vi "Motor_con.vi"(4 "Q_Process_Data_Err_IN":errorcluster caption="Q_Process_DATA_Err_IN", 6 "Q_Process_Data2_IN":refnum<queue>, 8 "Error_IN":errorcluster caption="error out", 9 "Notifier_IN":refnum<notifier>, 10 "Q_MotorCmd_Err_IN":errorcluster caption="에러 출력", 11 "Q_MotorCmd_IN":refnum<queue>) -> ()   [LabVIEW 2019]
uses:
  <vilib>/Platform/TimedLoop/XDataNode/timing_clust.ctl
  <vilib>/Platform/TimedLoop/XDataNode/nitl_modes.ctl
  <vilib>/Platform/TimedLoop/XDataNode/wakeup.ctl
  Type/SDO_Command.ctl
  CANopen/CANopen_SubVI/Controlword.ctl
  RT_GLOBAL.vi
  <vilib>/Platform/TimedLoop/XDataNode/XDataNode.xnode
  <vilib>/Platform/TimedLoop/XDataNode/XDNodeRunTimeDep.lvlib
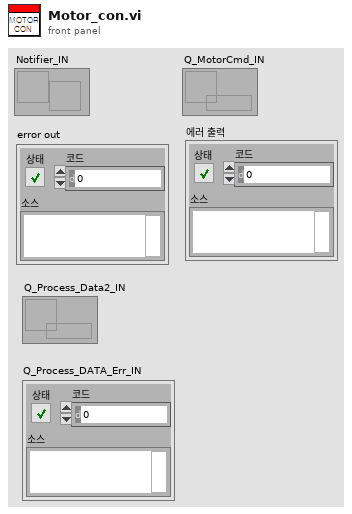
[diagram p1: front panel]
types:
  T1 = typedef "XDNodeRunTimeDep.lvlib/timing_clust.ctl" = cluster{"Expected End [f-1]":u64, "Actual End [f-1]":u64, "Finished Late? [f-1]":bool, "Expected End [i-1]":u64, "Actual End [i-1]":u64, "Finished Late? [i-1]":bool, "Expected Start [i]":u64, "Actual Start [i]":u64, "Expected Start [f]":u64, "Actual Start [f]":u64, "Source Name":string, "Structure Name":string, "Period":i64, "Deadline":i64, "Offset":i64, "Start":i64, "Priority":i32, "Timeout":i32, "Mode":T2, "Wakeup Reason":T3, "Error":errorcluster, "Source Type":string, "Secondary Source Type":string, "Global End Time":u64, "Global Start Time":u64, "Frame Duration":u64, "Iteration Duration":u64, "Assigned CPU":i32, "I/O Scan Engine Mode":u32}
  T2 = typedef "XDNodeRunTimeDep.lvlib/nitl_modes.ctl" = enum32{"No Change", "Process missed periods, maintain original phase", "Discard missed periods, maintain original phase", "Process missed periods, ignore original phase", "Discard missed periods, ignore original phase"}
  T3 = typedef "XDNodeRunTimeDep.lvlib/wakeup.ctl" = enum32{"Normal", "Aborted", "Asynchronous wakeup", "Timing source error", "Timed loop error", "Timeout"}
  T4 = cluster{"Target":i32, "Manual":u8[], "Velocity":u32, "Acc/Dec":u32}
  T5 = typedef "SDO_Command.ctl" = enum16{"Idle", "Shutdown", "Switch On", "Enable Operation", "Disable Voltage", "Quikstop", "Disable Operation", "Fault Reset", "Manual", "Statusword", "Mode of Operation", "Mode Display", "Target Position", "Position Actual Value", "Controlword_Move", "Profile Velocity", "Profile Acceleration", "Profile Deceleration", "Move"}
  T6 = typedef "CANFrameControl.ctl" = cluster{"identifier":u32, "extended?":bool, "type":u8, "payload":u8[]}
  T7 = cluster{"Cmd":string, "Data1":variant, "Data2":variant}
  T8 = typedef "Controlword.ctl" = u8
  T9 = cluster{"[0]":bool, "[1]":bool, "[2]":bool, "[3]":bool, "[4]":bool, "[5]":bool, "[6]":bool, "[7]":bool, "[8]":bool, "[9]":bool, "[10]":bool, "[11]":bool, "[12]":bool, "[13]":bool, "[14]":bool, "[15]":bool}
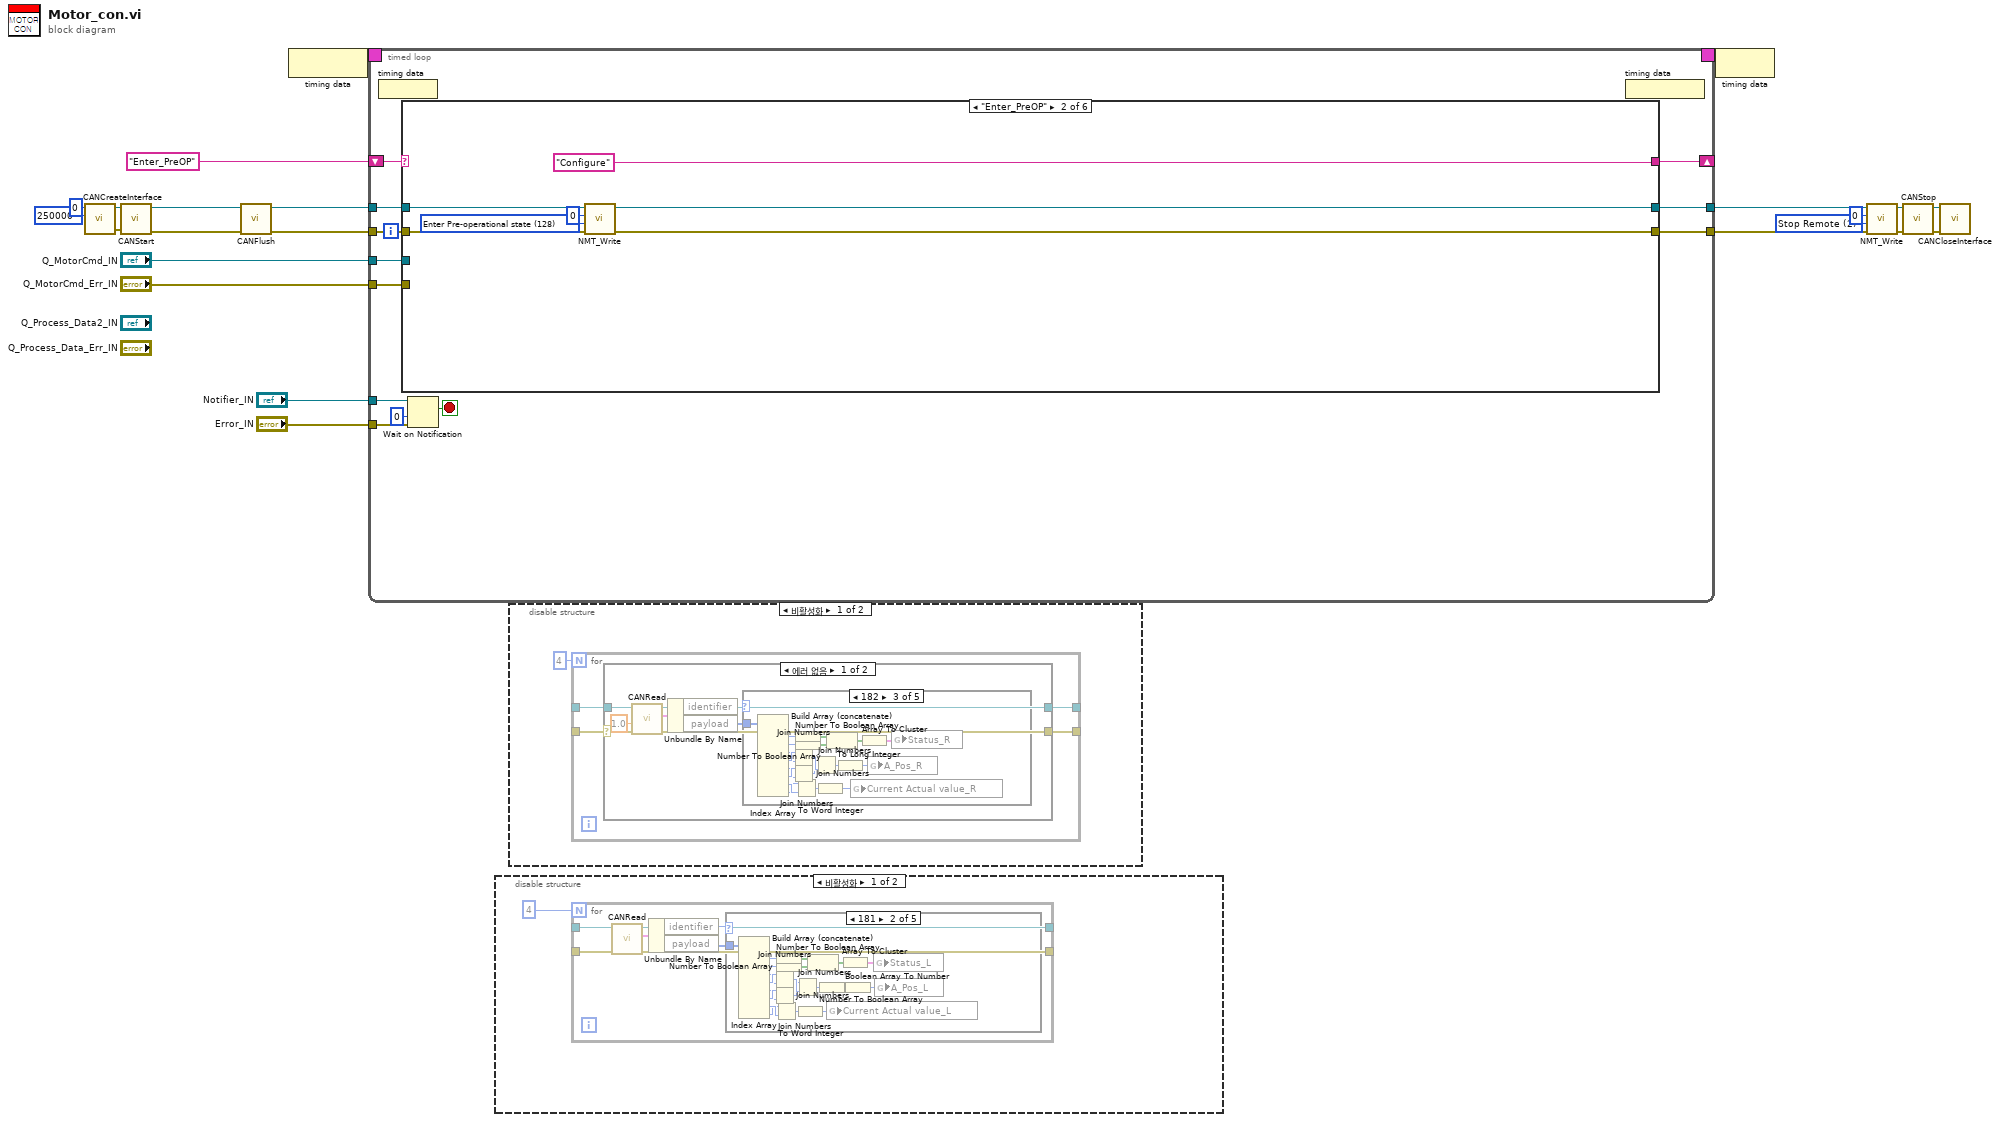
[diagram p0: block diagram]
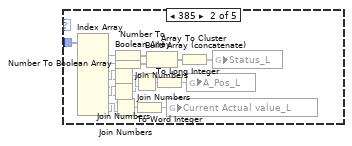
[diagram p3: hidden frame]
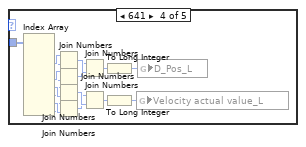
[diagram p4: hidden frame]
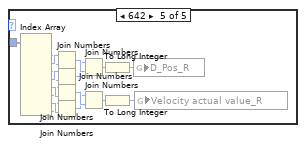
[diagram p5: hidden frame]
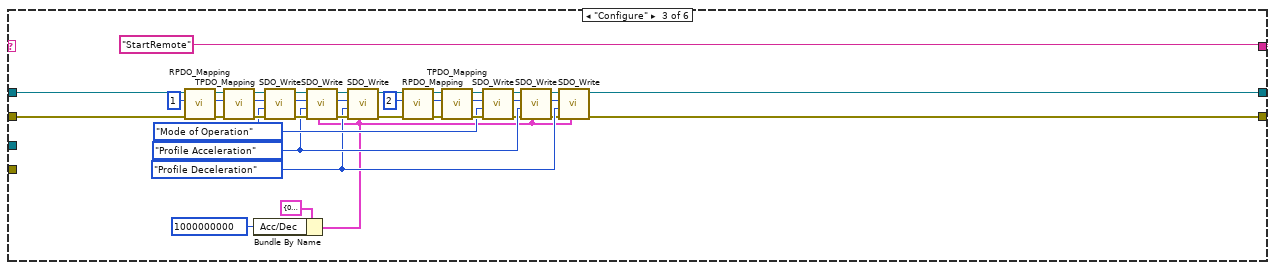
[diagram p9: hidden frame]
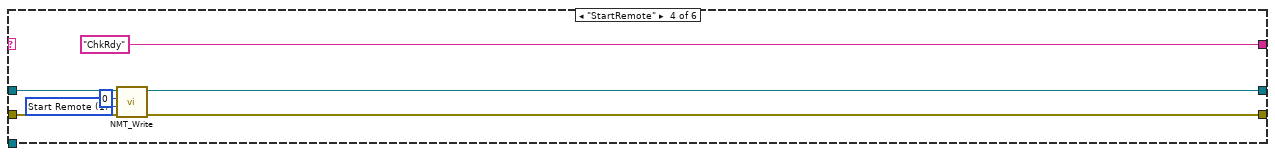
[diagram p10: hidden frame]
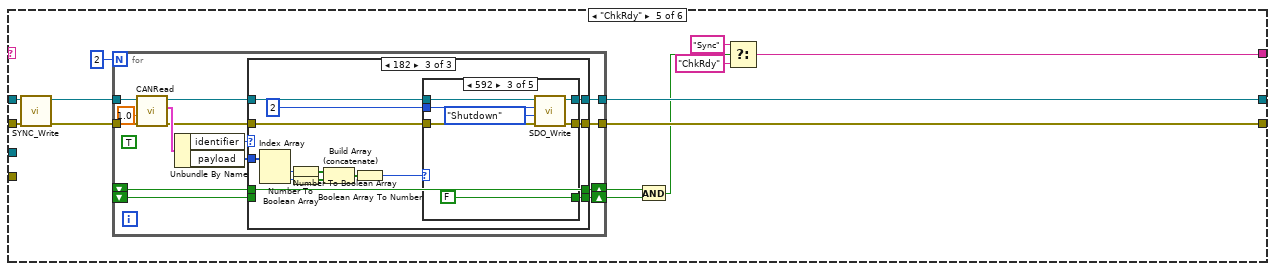
[diagram p11: hidden frame]
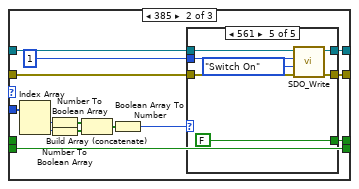
[diagram p13: hidden frame]
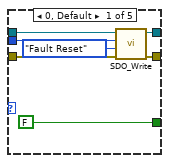
[diagram p14: hidden frame]
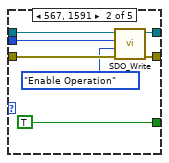
[diagram p15: hidden frame]
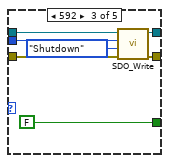
[diagram p16: hidden frame]
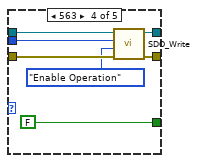
[diagram p17: hidden frame]
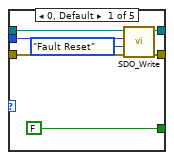
[diagram p18: hidden frame]
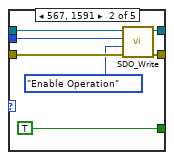
[diagram p19: hidden frame]
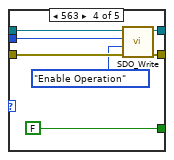
[diagram p20: hidden frame]
diagram:
  w15 = u8 2 items=["Start Remote"=1, "Stop Remote"=2, "Enter Pre-operational state"=128, "Reset node"=129, "Reset communication"=130] ("Command")
  n1 = call <vilib>:"CANCreateInterface.vi"("baud rate (125000 bps)"=u32 250000, "interface index"=u32 0) -> ("error out"=w8:errorcluster, "interface object out"=w9:refnum<k20>)  [unwired: 8 in]
  n2 = call <vilib>:"CANStart.vi"("error in (no error)"=w8, "interface object in"=w9) -> ("error out"=w3:errorcluster, "interface object out"=w4:refnum<k20>)  [unwired: 8 in]
  n3 = call <vilib>:"CANFlush.vi"("error in (no error)"=w3, "interface object in"=w4) -> ("error out"=w1:errorcluster, "interface object out"=w2:refnum<k20>)  [unwired: 8 in]
  n4 = node-c288() -> (w12:T1)
  n5 = timed-loop {
    shift-right: [w35] -> _
    shift-left: "Enter_PreOP" -> [w34]
    tunnel: "Q_MotorCmd_IN" -> [w32]
    tunnel: "Q_MotorCmd_Err_IN" -> [w31]
    tunnel: [w33] -> w23
    timing: w12 -> [_]
    timing-out: [_] -> w11
    tunnel: w1 -> [w29]
    tunnel: "Notifier_IN" -> [w25]
    tunnel: "Error_IN" -> [w24]
    tunnel: w2 -> [w28]
    tunnel: [w30] -> w17
    stop <- w27 stop-if-true
    n6 = node-c288() -> ()  [unwired: 1 in]
    n7 = case shown="\"Enter_PreOP\"" w34 {
      selector: w34 -> [w40 _ _ _ _ w219]
      tunnel: [w40 "Configure" "StartRemote" "ChkRdy" w88 w220] -> w35
      tunnel: [w39 w42 w49 w80 w92 w221] -> w30
      tunnel: w28 -> [w39 w45 w52 w83 w94 w223]
      tunnel: [w38 w41 w48 w79 w91 w215] -> w33
      tunnel: w29 -> [w38 w44 w51 w82 w93 w222]
      tunnel: w32 -> [_ _ _ _ _ w230]
      tunnel: w31 -> [_ _ _ _ _ w229]
      frame "거짓", Default {
      }
      frame "Enter_PreOP" {
        w47 = u8 128 items=["Start Remote"=1, "Stop Remote"=2, "Enter Pre-operational state"=128, "Reset node"=129, "Reset communication"=130] ("Command")
        n8 = call "NMT_Write.vi"("error in"=w44, "Command"=w47, "Node_ID"=u32 0, "interface object in"=w45) -> ("error out"=w41:errorcluster, "interface object out"=w42:refnum<k20>)  [unwired: 6 in]
      }
      frame "Configure" {
        w56 = SDO_Command."Profile Deceleration" ("Command")
        w57 = SDO_Command."Profile Acceleration" ("Command")
        w58 = u32 2 ("Node_ID")
        w69 = u32 1 ("Node_ID")
        w61 = SDO_Command."Mode of Operation" ("Command")
        n9 = call "RPDO_Mapping.vi"("error in"=w51, "Node_ID"=w69, "interface object in"=w52) -> ("error out"=w77:errorcluster, "interface object out"=w78:refnum<k20>)  [unwired: 7 in]
        n10 = call "TPDO_Mapping.vi"("error in"=w77, "Node_ID"=w69, "interface object in"=w78) -> ("error out"=w75:errorcluster, "interface object out"=w76:refnum<k20>)  [unwired: 7 in]
        n11 = Bundle By Name(cluster=T4 {"Target"=0, "Manual"=[], "Velocity"=0, "Acc/Dec"=0} ("Parameter"), "Acc/Dec"=u32 1000000000) -> (w55:T4)
        n12 = call "SDO_Write.vi"("error in"=w75, "Command"=w61, "Node_ID"=w69, "interface object in"=w76) -> ("error out"=w68:errorcluster, "interface object out"=w67:refnum<k20>)  [unwired: 6 in]
        n13 = call "SDO_Write.vi"("Parameter"=w55, "error in"=w68, "Command"=w57, "Node_ID"=w69, "interface object in"=w67) -> ("error out"=w66:errorcluster, "interface object out"=w70:refnum<k20>)  [unwired: 5 in]
        n14 = call "SDO_Write.vi"("Parameter"=w55, "error in"=w66, "Command"=w56, "Node_ID"=w69, "interface object in"=w70) -> ("error out"=w62:errorcluster, "interface object out"=w63:refnum<k20>)  [unwired: 5 in]
        n15 = call "RPDO_Mapping.vi"("error in"=w62, "Node_ID"=w58, "interface object in"=w63) -> ("error out"=w73:errorcluster, "interface object out"=w74:refnum<k20>)  [unwired: 7 in]
        n16 = call "TPDO_Mapping.vi"("error in"=w73, "Node_ID"=w58, "interface object in"=w74) -> ("error out"=w71:errorcluster, "interface object out"=w72:refnum<k20>)  [unwired: 7 in]
        n17 = call "SDO_Write.vi"("error in"=w71, "Command"=w61, "Node_ID"=w58, "interface object in"=w72) -> ("error out"=w54:errorcluster, "interface object out"=w60:refnum<k20>)  [unwired: 6 in]
        n18 = call "SDO_Write.vi"("Parameter"=w55, "error in"=w54, "Command"=w57, "Node_ID"=w58, "interface object in"=w60) -> ("error out"=w53:errorcluster, "interface object out"=w59:refnum<k20>)  [unwired: 5 in]
        n19 = call "SDO_Write.vi"("Parameter"=w55, "error in"=w53, "Command"=w56, "Node_ID"=w58, "interface object in"=w59) -> ("error out"=w48:errorcluster, "interface object out"=w49:refnum<k20>)  [unwired: 5 in]
      }
      frame "StartRemote" {
        w84 = u8 1 items=["Start Remote"=1, "Stop Remote"=2, "Enter Pre-operational state"=128, "Reset node"=129, "Reset communication"=130] ("Command")
        n20 = call "NMT_Write.vi"("error in"=w82, "Command"=w84, "Node_ID"=u32 0, "interface object in"=w83) -> ("error out"=w79:errorcluster, "interface object out"=w80:refnum<k20>)  [unwired: 6 in]
      }
      frame "ChkRdy" {
        n21 = call "SYNC_Write.vi"("error in"=w93, "interface object in"=w94) -> ("error out"=w96:errorcluster, "interface object out"=w97:refnum<k20>)  [unwired: 8 in]
        n22 = for {
          N: 2 -> [_]
          tunnel: w97 -> [w107]
          tunnel: [w104] -> w92
          tunnel: w96 -> [w106]
          tunnel: [w103] -> w91
          shift-right: [w102] -> w90
          shift-left: _ -> [w100]
          shift-right: [w101] -> w89
          shift-left: _ -> [w99]
          (unwired) TRUE
          n23 = call <vilib>:"CANRead.vi"("error in (no error)"=w106, "timeout (0 s)"=1.0, "interface object in"=w107) -> ("error out"=w108:errorcluster, "CAN frame"=w112:T6, "interface object out"=w109:refnum<k20>)  [unwired: 5 in, 1 out]
          n24 = Unbundle By Name(w112) -> ("identifier"=w111:u32, "payload"=w110:u8[])
          n25 = case shown="182" w111 {
            tunnel: w110 -> [_ w125 w174]
            tunnel: w109 -> [w115 w124 w171]
            tunnel: w108 -> [w116 w123 w170]
            tunnel: [w116 w122 w172] -> w103
            tunnel: [w115 w121 w173] -> w104
            tunnel: [w114 w119 w166] -> w102
            tunnel: [w113 w117 w168] -> w101
            tunnel: w100 -> [w114 _ w166]
            tunnel: w99 -> [w113 w117 _]
            frame 0, Default {
            }
            frame 385 {
              n26 = Index Array(array=w125) -> (element #1=w130:u8, element #2=w129:u8)  [unwired: 2 in]
              n27 = Number To Boolean Array(number=w130) -> (Boolean array=w128:bool[])
              n28 = Number To Boolean Array(number=w129) -> (Boolean array=w127:bool[])
              n29 = Build Array (concatenate)(w128, w127) -> (w126:bool[])
              n30 = Boolean Array To Number(Boolean array=w126) -> (number=w120:u32)
              n31 = case shown="561" w120 {
                tunnel: u32 1 -> [w135 w142 w149 w156 w163]
                tunnel: w124 -> [w136 w143 w150 w155 w164]
                tunnel: w123 -> [w134 w141 w148 w157 w162]
                tunnel: [FALSE TRUE FALSE FALSE FALSE] -> w119
                tunnel: [w132 w140 w146 w154 w161] -> w121
                tunnel: [w133 w139 w147 w153 w160] -> w122
                frame 0, Default {
                  n32 = call "SDO_Write.vi"("error in"=w134, "Command"=SDO_Command."Fault Reset", "Node_ID"=w135, "interface object in"=w136) -> ("error out"=w133:errorcluster, "interface object out"=w132:refnum<k20>)  [unwired: 6 in]
                }
                frame 567, 1591 {
                  n33 = call "SDO_Write.vi"("error in"=w141, "Command"=SDO_Command."Enable Operation", "Node_ID"=w142, "interface object in"=w143) -> ("error out"=w139:errorcluster, "interface object out"=w140:refnum<k20>)  [unwired: 6 in]
                }
                frame 592 {
                  n34 = call "SDO_Write.vi"("error in"=w148, "Command"=SDO_Command."Shutdown", "Node_ID"=w149, "interface object in"=w150) -> ("error out"=w147:errorcluster, "interface object out"=w146:refnum<k20>)  [unwired: 6 in]
                }
                frame 563 {
                  n35 = call "SDO_Write.vi"("error in"=w157, "Command"=SDO_Command."Enable Operation", "Node_ID"=w156, "interface object in"=w155) -> ("error out"=w153:errorcluster, "interface object out"=w154:refnum<k20>)  [unwired: 6 in]
                }
                frame 561 {
                  n36 = call "SDO_Write.vi"("error in"=w162, "Command"=SDO_Command."Switch On", "Node_ID"=w163, "interface object in"=w164) -> ("error out"=w160:errorcluster, "interface object out"=w161:refnum<k20>)  [unwired: 6 in]
                }
              }
            }
            frame 386 {
              n37 = Index Array(array=w174) -> (element #1=w179:u8, element #2=w178:u8)  [unwired: 2 in]
              n38 = Number To Boolean Array(number=w179) -> (Boolean array=w177:bool[])
              n39 = Number To Boolean Array(number=w178) -> (Boolean array=w176:bool[])
              n40 = Build Array (concatenate)(w177, w176) -> (w175:bool[])
              n41 = Boolean Array To Number(Boolean array=w175) -> (number=w169:u32)
              n42 = case shown="592" w169 {
                tunnel: u32 2 -> [w184 w190 w198 w205 w212]
                tunnel: w171 -> [w185 w191 w199 w206 w213]
                tunnel: w170 -> [w183 w192 w197 w204 w211]
                tunnel: [FALSE TRUE FALSE FALSE FALSE] -> w168
                tunnel: [w182 w189 w196 w203 w210] -> w173
                tunnel: [w181 w188 w195 w202 w209] -> w172
                frame 0, Default {
                  n43 = call "SDO_Write.vi"("error in"=w183, "Command"=SDO_Command."Fault Reset", "Node_ID"=w184, "interface object in"=w185) -> ("error out"=w181:errorcluster, "interface object out"=w182:refnum<k20>)  [unwired: 6 in]
                }
                frame 567, 1591 {
                  n44 = call "SDO_Write.vi"("error in"=w192, "Command"=SDO_Command."Enable Operation", "Node_ID"=w190, "interface object in"=w191) -> ("error out"=w188:errorcluster, "interface object out"=w189:refnum<k20>)  [unwired: 6 in]
                }
                frame 592 {
                  n45 = call "SDO_Write.vi"("error in"=w197, "Command"=SDO_Command."Shutdown", "Node_ID"=w198, "interface object in"=w199) -> ("error out"=w195:errorcluster, "interface object out"=w196:refnum<k20>)  [unwired: 6 in]
                }
                frame 563 {
                  n46 = call "SDO_Write.vi"("error in"=w204, "Command"=SDO_Command."Enable Operation", "Node_ID"=w205, "interface object in"=w206) -> ("error out"=w202:errorcluster, "interface object out"=w203:refnum<k20>)  [unwired: 6 in]
                }
                frame 561 {
                  n47 = call "SDO_Write.vi"("error in"=w211, "Command"=SDO_Command."Switch On", "Node_ID"=w212, "interface object in"=w213) -> ("error out"=w209:errorcluster, "interface object out"=w210:refnum<k20>)  [unwired: 6 in]
                }
              }
            }
          }
        }
        n48 = And(x=w90, y=w89) -> (x .and. y?=w86:bool)
        n49 = Select(t="Sync", s=w86, f="ChkRdy") -> (s? t:f=w88:string)
      }
      frame "Sync" {
        n50 = Dequeue Element(queue=w230, timeout in ms (-1)=0 ("타임아웃(ms) (-1)"), error in (no error)=w229) -> (element=w227:T7, timed out?=w228:bool)  [unwired: 2 out]
        n51 = case shown="거짓" w228 {
          tunnel: w227 -> [w320 _]
          tunnel: w222 -> [w317 w499]
          tunnel: w223 -> [w316 w500]
          tunnel: [w315 w500] -> w226
          tunnel: [w314 w499] -> w225
          tunnel: [w312 w498] -> w220
          tunnel: w219 -> [w311 w498]
          frame False {
            n52 = Unbundle By Name(w320) -> ("Cmd"=w319:string, "Data1"=w318:variant, "Data2"=w313:variant)
            n53 = case shown="\"Set_Vel_Pos\"" w319 {
              tunnel: w318 -> [_ w330 w368 w412 w448 w476 _]
              tunnel: w317 -> [w322 w336 w358 w410 w444 w471 w496]
              tunnel: w316 -> [w323 w338 w359 w409 w446 w472 w497]
              tunnel: [w323 w337 w361 w405 w445 w467 w492] -> w315
              tunnel: [w322 w335 w360 w406 w443 w468 w491] -> w314
              tunnel: w313 -> [_ _ w362 _ _ _ _]
              tunnel: [w321 w324 w354 w403 w437 w466 "ChkRdy"] -> w312
              tunnel: w311 -> [w321 w324 w354 w403 w437 w466 _]
              frame "거짓", Default {
              }
              frame "Set_Vel" {
                n54 = Variant To Data(type=u32[] [], Variant=w330) -> (data=w333:u32[])  [unwired: 1 in, 1 out]
                n55 = Index Array(array=w333) -> (element #1=w332:u32, element #2=w331:u32)  [unwired: 2 in]
                n56 = Bundle By Name(cluster=T4 {"Target"=0, "Manual"=[], "Velocity"=0, "Acc/Dec"=0} ("Parameter"), "Velocity"=w332, "Acc/Dec"=w331) -> (w326:T4)
                n57 = for {
                  N: 2 -> [_]
                  tunnel: w338 -> [w343]
                  tunnel: [w350] -> w337
                  tunnel: w336 -> [w342]
                  tunnel: [w349] -> w335
                  tunnel: w326 -> [w348]
                  tunnel: SDO_Command."Profile Deceleration" ("Command") -> [w347]
                  tunnel: SDO_Command."Profile Acceleration" ("Command") -> [w346]
                  tunnel: SDO_Command."Profile Velocity" ("Command") -> [w345]
                  i -> [w352]
                  n58 = Increment ("증가")(x=w352) -> (x+1=w344:u32)
                  n59 = call "SDO_Write.vi"("Parameter"=w348, "error in"=w342, "Command"=w345, "Node_ID"=w344, "interface object in"=w343) -> ("error out"=w353:errorcluster, "interface object out"=w351:refnum<k20>)  [unwired: 5 in]
                  n60 = call "SDO_Write.vi"("Parameter"=w348, "error in"=w353, "Command"=w346, "Node_ID"=w344, "interface object in"=w351) -> ("error out"=w341:errorcluster, "interface object out"=w340:refnum<k20>)  [unwired: 5 in]
                  n61 = call "SDO_Write.vi"("Parameter"=w348, "error in"=w341, "Command"=w347, "Node_ID"=w344, "interface object in"=w340) -> ("error out"=w349:errorcluster, "interface object out"=w350:refnum<k20>)  [unwired: 5 in]
                }
              }
              frame "Set_Vel_Pos" {
                w365 = T8 63 items=["Manual"=255, "Shutdown"=6, "Switch On & Disable"=7, "Enable Operation"=15, "Disable Voltage"=0, "Quikstop"=2, "Fault Reset"=128, "Move"=63] ("Controlword")
                n62 = Variant To Data(type=i32[] [], Variant=w362) -> (data=w367:i32[])  [unwired: 1 in, 1 out]
                n63 = Variant To Data(type=u32[] [], Variant=w368) -> (data=w372:u32[])  [unwired: 1 in, 1 out]
                n64 = Index Array(array=w367) -> (element #1=w355:i32, element #2=w364:i32)  [unwired: 2 in]
                n65 = Index Array(array=w372) -> (element #2=w370:u32)  [unwired: 2 in, 1 out]
                n66 = Bundle By Name(cluster=T4 {"Target"=0, "Manual"=[], "Velocity"=0, "Acc/Dec"=0} ("Parameter"), "Velocity"=w370) -> (w356:T4)
                n67 = case shown="2" w355 {
                  tunnel: [w374 w376 w390] -> w361
                  tunnel: [w373 w375 w389] -> w360
                  tunnel: w365 -> [_ w388 w402]
                  tunnel: w364 -> [_ w383 w397]
                  tunnel: SDO_Command."Enable Operation" ("Command") -> [_ w387 w401]
                  tunnel: w359 -> [w374 w380 w394]
                  tunnel: w358 -> [w373 w381 w395]
                  tunnel: SDO_Command."Profile Velocity" ("Command") -> [_ w382 w396]
                  tunnel: w356 -> [_ w384 w398]
                  frame 0, Default {
                  }
                  frame 1 {
                    w379 = u32 1 ("Node_ID")
                    n68 = call "SDO_Write.vi"("error in"=w381, "Command"=w387, "Node_ID"=w379, "interface object in"=w380) -> ("error out"=w377:errorcluster, "interface object out"=w378:refnum<k20>)  [unwired: 6 in]
                    n69 = call "SDO_Write.vi"("Parameter"=w384, "error in"=w377, "Command"=w382, "Node_ID"=w379, "interface object in"=w378) -> ("error out"=w385:errorcluster, "interface object out"=w386:refnum<k20>)  [unwired: 5 in]
                    n70 = call "RPDO_0x1600.vi"("Target Pos"=w383, "Controlword"=w388, "error in"=w385, "Node_ID"=w379, "interface object in"=w386) -> ("error out"=w375:errorcluster, "interface object out"=w376:refnum<k20>)  [unwired: 5 in]
                  }
                  frame 2 {
                    w393 = u32 2 ("Node_ID")
                    n71 = call "SDO_Write.vi"("error in"=w395, "Command"=w401, "Node_ID"=w393, "interface object in"=w394) -> ("error out"=w391:errorcluster, "interface object out"=w392:refnum<k20>)  [unwired: 6 in]
                    n72 = call "SDO_Write.vi"("Parameter"=w398, "error in"=w391, "Command"=w396, "Node_ID"=w393, "interface object in"=w392) -> ("error out"=w399:errorcluster, "interface object out"=w400:refnum<k20>)  [unwired: 5 in]
                    n73 = call "RPDO_0x1600.vi"("Target Pos"=w397, "Controlword"=w402, "error in"=w399, "Node_ID"=w393, "interface object in"=w400) -> ("error out"=w389:errorcluster, "interface object out"=w390:refnum<k20>)  [unwired: 5 in]
                  }
                }
              }
              frame "Set_Pos" {
                w408 = T8 63 items=["Manual"=255, "Shutdown"=6, "Switch On & Disable"=7, "Enable Operation"=15, "Disable Voltage"=0, "Quikstop"=2, "Fault Reset"=128, "Move"=63] ("Controlword")
                n74 = Variant To Data(type=i32[] [], Variant=w412) -> (data=w414:i32[])  [unwired: 1 in, 1 out]
                n75 = Index Array(array=w414) -> (element #1=w411:i32, element #2=w407:i32)  [unwired: 2 in]
                n76 = case shown="1" w411 {
                  tunnel: w410 -> [w421 w425 w435]
                  tunnel: w409 -> [w422 w426 w434]
                  tunnel: [w416 w426 w431] -> w405
                  tunnel: [w415 w425 w430] -> w406
                  tunnel: w408 -> [w424 _ w436]
                  tunnel: w407 -> [w423 _ w427]
                  tunnel: SDO_Command."Enable Operation" ("Command") -> [w418 _ w429]
                  frame 2 {
                    w419 = u32 2 ("Node_ID")
                    n77 = call "RPDO_0x1600.vi"("Target Pos"=w423, "Controlword"=w424, "error in"=w421, "Node_ID"=w419, "interface object in"=w422) -> ("error out"=w417:errorcluster, "interface object out"=w420:refnum<k20>)  [unwired: 5 in]
                    n78 = call "SDO_Write.vi"("error in"=w417, "Command"=w418, "Node_ID"=w419, "interface object in"=w420) -> ("error out"=w415:errorcluster, "interface object out"=w416:refnum<k20>)  [unwired: 6 in]
                  }
                  frame 0, Default {
                  }
                  frame 1 {
                    w428 = u32 1 ("Node_ID")
                    n79 = call "RPDO_0x1600.vi"("Target Pos"=w427, "Controlword"=w436, "error in"=w435, "Node_ID"=w428, "interface object in"=w434) -> ("error out"=w432:errorcluster, "interface object out"=w433:refnum<k20>)  [unwired: 5 in]
                    n80 = call "SDO_Write.vi"("error in"=w432, "Command"=w429, "Node_ID"=w428, "interface object in"=w433) -> ("error out"=w430:errorcluster, "interface object out"=w431:refnum<k20>)  [unwired: 6 in]
                  }
                }
              }
              frame "Set_Vel_Each" {
                n81 = Variant To Data(type=u32[] [], Variant=w448) -> (data=w449:u32[])  [unwired: 1 in, 1 out]
                n82 = Index Array(array=w449) -> (element #1=w447:u32, element #2=w441:u32)  [unwired: 2 in]
                n83 = Bundle By Name(cluster=T4 {"Target"=0, "Manual"=[], "Velocity"=0, "Acc/Dec"=0} ("Parameter"), "Velocity"=w441) -> (w440:T4)
                n84 = case shown="1" w447 {
                  tunnel: w446 -> [w451 w453 w460]
                  tunnel: [w451 w457 w461] -> w445
                  tunnel: w444 -> [w450 w454 w459]
                  tunnel: [w450 w458 w465] -> w443
                  tunnel: w440 -> [_ w452 w464]
                  tunnel: SDO_Command."Profile Velocity" ("Command") -> [_ w455 w462]
                  frame 0, Default {
                  }
                  frame 1 {
                    n85 = call "SDO_Write.vi"("Parameter"=w452, "error in"=w454, "Command"=w455, "Node_ID"=u32 1, "interface object in"=w453) -> ("error out"=w458:errorcluster, "interface object out"=w457:refnum<k20>)  [unwired: 5 in]
                  }
                  frame 2 {
                    n86 = call "SDO_Write.vi"("Parameter"=w464, "error in"=w459, "Command"=w462, "Node_ID"=u32 2, "interface object in"=w460) -> ("error out"=w465:errorcluster, "interface object out"=w461:refnum<k20>)  [unwired: 5 in]
                  }
                }
              }
              frame "Set_Pos_All" {
                w473 = T8 63 items=["Manual"=255, "Shutdown"=6, "Switch On & Disable"=7, "Enable Operation"=15, "Disable Voltage"=0, "Quikstop"=2, "Fault Reset"=128, "Move"=63] ("Controlword")
                n87 = Variant To Data(type=0, Variant=w476) -> (data=w474:i32)  [unwired: 1 in, 1 out]
                n88 = for {
                  N: 2 -> [_]
                  tunnel: w474 -> [w487]
                  tunnel: w473 -> [w486]
                  tunnel: w472 -> [w480]
                  tunnel: w471 -> [w479]
                  tunnel: SDO_Command."Enable Operation" ("Command") -> [w483]
                  tunnel: [w477] -> w468
                  tunnel: [w478] -> w467
                  i -> [w485]
                  n89 = Increment ("증가")(x=w485) -> (x+1=w484:u32)
                  n90 = call "SDO_Write.vi"("error in"=w479, "Command"=w483, "Node_ID"=w484, "interface object in"=w480) -> ("error out"=w481:errorcluster, "interface object out"=w482:refnum<k20>)  [unwired: 6 in]
                  n91 = call "RPDO_0x1600.vi"("Target Pos"=w487, "Controlword"=w486, "error in"=w481, "Node_ID"=w484, "interface object in"=w482) -> ("error out"=w477:errorcluster, "interface object out"=w478:refnum<k20>)  [unwired: 5 in]
                }
              }
              frame "Stop" {
                w489 = T8 2 items=["Manual"=255, "Shutdown"=6, "Switch On & Disable"=7, "Enable Operation"=15, "Disable Voltage"=0, "Quikstop"=2, "Fault Reset"=128, "Move"=63] ("Controlword")
                n92 = call "RPDO_0x1600.vi"("Controlword"=w489, "error in"=w496, "Node_ID"=u32 1, "interface object in"=w497) -> ("error out"=w493:errorcluster, "interface object out"=w494:refnum<k20>)  [unwired: 6 in]
                n93 = call "RPDO_0x1600.vi"("Controlword"=w489, "error in"=w493, "Node_ID"=u32 2, "interface object in"=w494) -> ("error out"=w491:errorcluster, "interface object out"=w492:refnum<k20>)  [unwired: 6 in]
              }
            }
          }
          frame True {
          }
        }
        n94 = call "SYNC_Write.vi"("error in"=w225, "interface object in"=w226) -> ("error out"=w217:errorcluster, "interface object out"=w218:refnum<k20>)  [unwired: 8 in]
        n95 = for {
          N: 4 -> [_]
          tunnel: w217 -> [w234]
          tunnel: [w232] -> w215
          tunnel: w218 -> [w233]
          tunnel: [w238] -> w221
          n96 = call <vilib>:"CANRead.vi"("error in (no error)"=w234, "timeout (0 s)"=1.0, "interface object in"=w233) -> ("error out"=w232:errorcluster, "CAN frame"=w237:T6, "interface object out"=w238:refnum<k20>)  [unwired: 5 in, 1 out]
          n97 = Unbundle By Name(w237) -> ("identifier"=w236:u32, "payload"=w235:u8[])
          n98 = case shown="181" w236 {
            tunnel: w235 -> [_ w246 w265 w287 w298]
            frame 0, Default {
            }
            frame 385 {
              n99 = Index Array(array=w246) -> (element #1=w257:u8, element #2=w256:u8, element #3=w249:u8, element #4=w251:u8, element #5=w248:u8, element #6=w250:u8, element #7=w245:u8, element #8=w244:u8)  [unwired: 8 in]
              n100 = Join Numbers(hi=w251, lo=w249) -> ((hi.lo)=w252:u16)
              n101 = Join Numbers(hi=w250, lo=w248) -> ((hi.lo)=w247:u16)
              n102 = Join Numbers(hi=w244, lo=w245) -> ((hi.lo)=w243:u16)
              n103 = Number To Boolean Array(number=w257) -> (Boolean array=w255:bool[])
              n104 = Number To Boolean Array(number=w256) -> (Boolean array=w254:bool[])
              n105 = Join Numbers(hi=w247, lo=w252) -> ((hi.lo)=w242:u32)
              n106 = To Word Integer(number=w243) -> (16bit integer=w239:i16)
              n107 = Build Array (concatenate)(w255, w254) -> (w253:bool[])
              n108 = To Long Integer(number=w242) -> (32bit integer=w240:i32)
              n109 = global write "RT_GLOBAL.vi" "Current Actual value_L"(w239) -> ()
              n110 = Array To Cluster(array=w253) -> (cluster=w241:T9)
              n111 = global write "RT_GLOBAL.vi" "A_Pos_L"(w240) -> ()
              n112 = global write "RT_GLOBAL.vi" "Status_L"(w241) -> ()
            }
            frame 386 {
              n113 = Index Array(array=w265) -> (element #1=w276:u8, element #2=w275:u8, element #3=w268:u8, element #4=w270:u8, element #5=w267:u8, element #6=w269:u8, element #7=w264:u8, element #8=w263:u8)  [unwired: 8 in]
              n114 = Join Numbers(hi=w270, lo=w268) -> ((hi.lo)=w271:u16)
              n115 = Join Numbers(hi=w269, lo=w267) -> ((hi.lo)=w266:u16)
              n116 = Join Numbers(hi=w263, lo=w264) -> ((hi.lo)=w262:u16)
              n117 = Number To Boolean Array(number=w276) -> (Boolean array=w274:bool[])
              n118 = Number To Boolean Array(number=w275) -> (Boolean array=w273:bool[])
              n119 = Join Numbers(hi=w266, lo=w271) -> ((hi.lo)=w260:u32)
              n120 = To Word Integer(number=w262) -> (16bit integer=w258:i16)
              n121 = Build Array (concatenate)(w274, w273) -> (w272:bool[])
              n122 = To Long Integer(number=w260) -> (32bit integer=w259:i32)
              n123 = global write "RT_GLOBAL.vi" "Current Actual value_R"(w258) -> ()
              n124 = Array To Cluster(array=w272) -> (cluster=w261:T9)
              n125 = global write "RT_GLOBAL.vi" "A_Pos_R"(w259) -> ()
              n126 = global write "RT_GLOBAL.vi" "Status_R"(w261) -> ()
            }
            frame 641 {
              n127 = Index Array(array=w287) -> (element #1=w290:u8, element #2=w292:u8, element #3=w289:u8, element #4=w291:u8, element #5=w284:u8, element #6=w283:u8, element #7=w282:u8, element #8=w281:u8)  [unwired: 8 in]
              n128 = Join Numbers(hi=w292, lo=w290) -> ((hi.lo)=w293:u16)
              n129 = Join Numbers(hi=w291, lo=w289) -> ((hi.lo)=w288:u16)
              n130 = Join Numbers(hi=w283, lo=w284) -> ((hi.lo)=w286:u16)
              n131 = Join Numbers(hi=w281, lo=w282) -> ((hi.lo)=w285:u16)
              n132 = Join Numbers(hi=w288, lo=w293) -> ((hi.lo)=w280:u32)
              n133 = Join Numbers(hi=w285, lo=w286) -> ((hi.lo)=w278:u32)
              n134 = To Long Integer(number=w280) -> (32bit integer=w279:i32)
              n135 = To Long Integer(number=w278) -> (32bit integer=w277:i32)
              n136 = global write "RT_GLOBAL.vi" "Velocity actual value_L"(w277) -> ()
              n137 = global write "RT_GLOBAL.vi" "D_Pos_L"(w279) -> ()
            }
            frame 642 {
              n138 = Index Array(array=w298) -> (element #1=w307:u8, element #2=w309:u8, element #3=w306:u8, element #4=w308:u8, element #5=w302:u8, element #6=w301:u8, element #7=w300:u8, element #8=w299:u8)  [unwired: 8 in]
              n139 = Join Numbers(hi=w309, lo=w307) -> ((hi.lo)=w310:u16)
              n140 = Join Numbers(hi=w308, lo=w306) -> ((hi.lo)=w305:u16)
              n141 = Join Numbers(hi=w301, lo=w302) -> ((hi.lo)=w304:u16)
              n142 = Join Numbers(hi=w299, lo=w300) -> ((hi.lo)=w303:u16)
              n143 = Join Numbers(hi=w305, lo=w310) -> ((hi.lo)=w296:u32)
              n144 = Join Numbers(hi=w303, lo=w304) -> ((hi.lo)=w295:u32)
              n145 = To Long Integer(number=w296) -> (32bit integer=w297:i32)
              n146 = To Long Integer(number=w295) -> (32bit integer=w294:i32)
              n147 = global write "RT_GLOBAL.vi" "D_Pos_R"(w297) -> ()
              n148 = global write "RT_GLOBAL.vi" "Velocity actual value_R"(w294) -> ()
            }
          }
        }
      }
    }
    n149 = Wait on Notification(notifier=w25, timeout in ms (-1)=0 ("타임아웃(ms) (-1)"), error in (no error)=w24) -> (notification=w27:bool)  [unwired: 1 in, 3 out]
    n150 = node-c288() -> ()  [unwired: 1 out]
  }
  n151 = disable-structure shown="비활성화" {
    frame Disabled {
      n152 = for {
        N: 4 -> [_]
        tunnel: _ -> [w505]
        tunnel: _ -> [w504]
        tunnel: [w503] -> _
        tunnel: [w502] -> _
        n153 = call <vilib>:"CANRead.vi"("error in (no error)"=w504, "interface object in"=w505) -> ("error out"=w503:errorcluster, "CAN frame"=w508:T6, "interface object out"=w502:refnum<k20>)  [unwired: 6 in, 1 out]
        n154 = Unbundle By Name(w508) -> ("identifier"=w507:u32, "payload"=w506:u8[])
        n155 = case shown="181" w507 {
          tunnel: w506 -> [_ w513 w535 w558 w568]
          frame 0, Default {
          }
          frame 385 {
            n156 = Index Array(array=w513) -> (element #1=w528:u8, element #2=w527:u8, element #3=w519:u8, element #4=w521:u8, element #5=w518:u8, element #6=w520:u8, element #7=w512:u8, element #8=w511:u8)  [unwired: 8 in]
            n157 = Join Numbers(hi=w521, lo=w519) -> ((hi.lo)=w522:u16)
            n158 = Join Numbers(hi=w520, lo=w518) -> ((hi.lo)=w517:u16)
            n159 = Join Numbers(hi=w511, lo=w512) -> ((hi.lo)=w510:u16)
            n160 = Number To Boolean Array(number=w528) -> (Boolean array=w526:bool[])
            n161 = Number To Boolean Array(number=w527) -> (Boolean array=w525:bool[])
            n162 = Join Numbers(hi=w517, lo=w522) -> ((hi.lo)=w516:u32)
            n163 = To Word Integer(number=w510) -> (16bit integer=w509:i16)
            n164 = Build Array (concatenate)(w526, w525) -> (w524:bool[])
            n165 = Number To Boolean Array(number=w516) -> (Boolean array=w523:bool[])
            n166 = global write "RT_GLOBAL.vi" "Current Actual value_L"(w509) -> ()
            n167 = Array To Cluster(array=w524) -> (cluster=w514:T9)
            n168 = Boolean Array To Number ("불리언 배열을 숫자로")(Boolean array=w523) -> (number=w515:i32)
            n169 = global write "RT_GLOBAL.vi" "Status_L"(w514) -> ()
            n170 = global write "RT_GLOBAL.vi" "A_Pos_L"(w515) -> ()
          }
          frame 386 {
            n171 = Index Array(array=w535) -> (element #1=w548:u8, element #2=w547:u8, element #3=w539:u8, element #4=w541:u8, element #5=w538:u8, element #6=w540:u8, element #7=w532:u8, element #8=w531:u8)  [unwired: 8 in]
            n172 = Join Numbers(hi=w541, lo=w539) -> ((hi.lo)=w542:u16)
            n173 = Join Numbers(hi=w540, lo=w538) -> ((hi.lo)=w537:u16)
            n174 = Join Numbers(hi=w531, lo=w532) -> ((hi.lo)=w529:u16)
            n175 = Number To Boolean Array(number=w548) -> (Boolean array=w546:bool[])
            n176 = Number To Boolean Array(number=w547) -> (Boolean array=w545:bool[])
            n177 = Join Numbers(hi=w537, lo=w542) -> ((hi.lo)=w536:u32)
            n178 = To Word Integer(number=w529) -> (16bit integer=w530:i16)
            n179 = Build Array (concatenate)(w546, w545) -> (w544:bool[])
            n180 = Number To Boolean Array(number=w536) -> (Boolean array=w543:bool[])
            n181 = global write "RT_GLOBAL.vi" "Current Actual value_R"(w530) -> ()
            n182 = Array To Cluster(array=w544) -> (cluster=w533:T9)
            n183 = Boolean Array To Number ("불리언 배열을 숫자로")(Boolean array=w543) -> (number=w534:i32)
            n184 = global write "RT_GLOBAL.vi" "Status_R"(w533) -> ()
            n185 = global write "RT_GLOBAL.vi" "A_Pos_R"(w534) -> ()
          }
          frame 641 {
            n186 = Index Array(array=w558) -> (element #1=w563:u8, element #2=w565:u8, element #3=w562:u8, element #4=w564:u8, element #5=w552:u8, element #6=w551:u8, element #7=w550:u8, element #8=w549:u8)  [unwired: 8 in]
            n187 = Join Numbers(hi=w551, lo=w552) -> ((hi.lo)=w556:u16)
            n188 = Join Numbers(hi=w549, lo=w550) -> ((hi.lo)=w555:u16)
            n189 = Join Numbers(hi=w565, lo=w563) -> ((hi.lo)=w566:u16)
            n190 = Join Numbers(hi=w564, lo=w562) -> ((hi.lo)=w561:u16)
            n191 = Join Numbers(hi=w555, lo=w556) -> ((hi.lo)=w554:u32)
            n192 = Join Numbers(hi=w561, lo=w566) -> ((hi.lo)=w560:u32)
            n193 = Number To Boolean Array(number=w554) -> (Boolean array=w557:bool[])
            n194 = Number To Boolean Array(number=w560) -> (Boolean array=w567:bool[])
            n195 = Boolean Array To Number ("불리언 배열을 숫자로")(Boolean array=w557) -> (number=w553:i32)
            n196 = Boolean Array To Number ("불리언 배열을 숫자로")(Boolean array=w567) -> (number=w559:i32)
            n197 = global write "RT_GLOBAL.vi" "Velocity actual value_L"(w553) -> ()
            n198 = global write "RT_GLOBAL.vi" "D_Pos_L"(w559) -> ()
          }
          frame 642 {
            n199 = Index Array(array=w568) -> (element #1=w582:u8, element #2=w584:u8, element #3=w581:u8, element #4=w583:u8, element #5=w572:u8, element #6=w571:u8, element #7=w570:u8, element #8=w569:u8)  [unwired: 8 in]
            n200 = Join Numbers(hi=w584, lo=w582) -> ((hi.lo)=w585:u16)
            n201 = Join Numbers(hi=w583, lo=w581) -> ((hi.lo)=w580:u16)
            n202 = Join Numbers(hi=w571, lo=w572) -> ((hi.lo)=w576:u16)
            n203 = Join Numbers(hi=w569, lo=w570) -> ((hi.lo)=w575:u16)
            n204 = Join Numbers(hi=w580, lo=w585) -> ((hi.lo)=w579:u32)
            n205 = Join Numbers(hi=w575, lo=w576) -> ((hi.lo)=w574:u32)
            n206 = Number To Boolean Array(number=w579) -> (Boolean array=w586:bool[])
            n207 = Number To Boolean Array(number=w574) -> (Boolean array=w577:bool[])
            n208 = Boolean Array To Number ("불리언 배열을 숫자로")(Boolean array=w586) -> (number=w578:i32)
            n209 = Boolean Array To Number ("불리언 배열을 숫자로")(Boolean array=w577) -> (number=w573:i32)
            n210 = global write "RT_GLOBAL.vi" "D_Pos_R"(w578) -> ()
            n211 = global write "RT_GLOBAL.vi" "Velocity actual value_R"(w573) -> ()
          }
        }
      }
    }
    frame Enabled {
    }
  }
  n212 = disable-structure shown="비활성화" {
    frame Disabled {
      n213 = for {
        N: 4 -> [_]
        tunnel: _ -> [w588]
        tunnel: [w591] -> _
        tunnel: _ -> [w589]
        tunnel: [w590] -> _
        n214 = case shown="에러 없음" w588 {
          selector: w588 -> [w593 w672]
          tunnel: [w599 w672] -> w591
          tunnel: [w598 w673] -> w590
          tunnel: w589 -> [w597 w673]
          frame No Error {
            n215 = call <vilib>:"CANRead.vi"("error in (no error)"=w593, "timeout (0 s)"=1.0, "interface object in"=w597) -> ("error out"=w599:errorcluster, "CAN frame"=w596:T6, "interface object out"=w598:refnum<k20>)  [unwired: 5 in, 1 out]
            n216 = Unbundle By Name(w596) -> ("identifier"=w595:u32, "payload"=w594:u8[])
            n217 = case shown="182" w595 {
              tunnel: w594 -> [_ w607 w626 w648 w659]
              frame 0, Default {
              }
              frame 385 {
                n218 = Index Array(array=w607) -> (element #1=w618:u8, element #2=w617:u8, element #3=w610:u8, element #4=w612:u8, element #5=w609:u8, element #6=w611:u8, element #7=w606:u8, element #8=w605:u8)  [unwired: 8 in]
                n219 = Join Numbers(hi=w612, lo=w610) -> ((hi.lo)=w613:u16)
                n220 = Join Numbers(hi=w611, lo=w609) -> ((hi.lo)=w608:u16)
                n221 = Join Numbers(hi=w605, lo=w606) -> ((hi.lo)=w604:u16)
                n222 = Number To Boolean Array(number=w618) -> (Boolean array=w616:bool[])
                n223 = Number To Boolean Array(number=w617) -> (Boolean array=w615:bool[])
                n224 = Join Numbers(hi=w608, lo=w613) -> ((hi.lo)=w603:u32)
                n225 = To Word Integer(number=w604) -> (16bit integer=w600:i16)
                n226 = Build Array (concatenate)(w616, w615) -> (w614:bool[])
                n227 = To Long Integer(number=w603) -> (32bit integer=w601:i32)
                n228 = global write "RT_GLOBAL.vi" "Current Actual value_L"(w600) -> ()
                n229 = Array To Cluster(array=w614) -> (cluster=w602:T9)
                n230 = global write "RT_GLOBAL.vi" "A_Pos_L"(w601) -> ()
                n231 = global write "RT_GLOBAL.vi" "Status_L"(w602) -> ()
              }
              frame 386 {
                n232 = Index Array(array=w626) -> (element #1=w637:u8, element #2=w636:u8, element #3=w629:u8, element #4=w631:u8, element #5=w628:u8, element #6=w630:u8, element #7=w625:u8, element #8=w624:u8)  [unwired: 8 in]
                n233 = Join Numbers(hi=w631, lo=w629) -> ((hi.lo)=w632:u16)
                n234 = Join Numbers(hi=w630, lo=w628) -> ((hi.lo)=w627:u16)
                n235 = Join Numbers(hi=w624, lo=w625) -> ((hi.lo)=w623:u16)
                n236 = Number To Boolean Array(number=w637) -> (Boolean array=w635:bool[])
                n237 = Number To Boolean Array(number=w636) -> (Boolean array=w634:bool[])
                n238 = Join Numbers(hi=w627, lo=w632) -> ((hi.lo)=w621:u32)
                n239 = To Word Integer(number=w623) -> (16bit integer=w619:i16)
                n240 = Build Array (concatenate)(w635, w634) -> (w633:bool[])
                n241 = To Long Integer(number=w621) -> (32bit integer=w620:i32)
                n242 = global write "RT_GLOBAL.vi" "Current Actual value_R"(w619) -> ()
                n243 = Array To Cluster(array=w633) -> (cluster=w622:T9)
                n244 = global write "RT_GLOBAL.vi" "A_Pos_R"(w620) -> ()
                n245 = global write "RT_GLOBAL.vi" "Status_R"(w622) -> ()
              }
              frame 641 {
                n246 = Index Array(array=w648) -> (element #1=w651:u8, element #2=w653:u8, element #3=w650:u8, element #4=w652:u8, element #5=w645:u8, element #6=w644:u8, element #7=w643:u8, element #8=w642:u8)  [unwired: 8 in]
                n247 = Join Numbers(hi=w653, lo=w651) -> ((hi.lo)=w654:u16)
                n248 = Join Numbers(hi=w652, lo=w650) -> ((hi.lo)=w649:u16)
                n249 = Join Numbers(hi=w644, lo=w645) -> ((hi.lo)=w647:u16)
                n250 = Join Numbers(hi=w642, lo=w643) -> ((hi.lo)=w646:u16)
                n251 = Join Numbers(hi=w649, lo=w654) -> ((hi.lo)=w641:u32)
                n252 = Join Numbers(hi=w646, lo=w647) -> ((hi.lo)=w639:u32)
                n253 = To Long Integer(number=w641) -> (32bit integer=w640:i32)
                n254 = To Long Integer(number=w639) -> (32bit integer=w638:i32)
                n255 = global write "RT_GLOBAL.vi" "Velocity actual value_L"(w638) -> ()
                n256 = global write "RT_GLOBAL.vi" "D_Pos_L"(w640) -> ()
              }
              frame 642 {
                n257 = Index Array(array=w659) -> (element #1=w668:u8, element #2=w670:u8, element #3=w667:u8, element #4=w669:u8, element #5=w663:u8, element #6=w662:u8, element #7=w661:u8, element #8=w660:u8)  [unwired: 8 in]
                n258 = Join Numbers(hi=w670, lo=w668) -> ((hi.lo)=w671:u16)
                n259 = Join Numbers(hi=w669, lo=w667) -> ((hi.lo)=w666:u16)
                n260 = Join Numbers(hi=w662, lo=w663) -> ((hi.lo)=w665:u16)
                n261 = Join Numbers(hi=w660, lo=w661) -> ((hi.lo)=w664:u16)
                n262 = Join Numbers(hi=w666, lo=w671) -> ((hi.lo)=w657:u32)
                n263 = Join Numbers(hi=w664, lo=w665) -> ((hi.lo)=w656:u32)
                n264 = To Long Integer(number=w657) -> (32bit integer=w658:i32)
                n265 = To Long Integer(number=w656) -> (32bit integer=w655:i32)
                n266 = global write "RT_GLOBAL.vi" "D_Pos_R"(w658) -> ()
                n267 = global write "RT_GLOBAL.vi" "Velocity actual value_R"(w655) -> ()
              }
            }
          }
          frame Error {
          }
        }
      }
    }
    frame Enabled {
    }
  }
  n268 = node-c288(w11) -> ()
  n269 = call "NMT_Write.vi"("error in"=w23, "Command"=w15, "Node_ID"=u32 0, "interface object in"=w17) -> ("error out"=w19:errorcluster, "interface object out"=w20:refnum<k20>)  [unwired: 6 in]
  n270 = call <vilib>:"CANStop.vi"("error in (no error)"=w19, "interface object in"=w20) -> ("error out"=w22:errorcluster, "interface object out"=w21:refnum<k20>)  [unwired: 8 in]
  n271 = call <vilib>:"CANCloseInterface.vi"("error in (no error)"=w22, "interface object in"=w21) -> ()  [unwired: 9 in, 1 out]
